vi "Check_Connectivity_111-11_with_101_Subtracks-1.vi"(4 "[IN] Index of connected tracks \nwith \"101\" problem dot":i32[](array[numeric]), 6 "[IN] Index of connected tracks \nwith \"111\" or \"11\" problem dot":i32[](array[numeric])) -> (1 "[OUT] Tracks aren't \nconnected after \"101\"":bool)   [LabVIEW 2013]
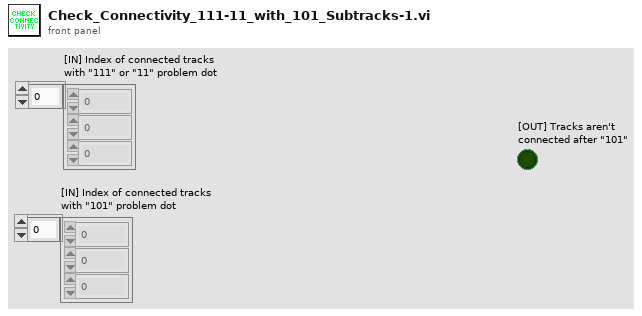
[diagram p1: front panel]
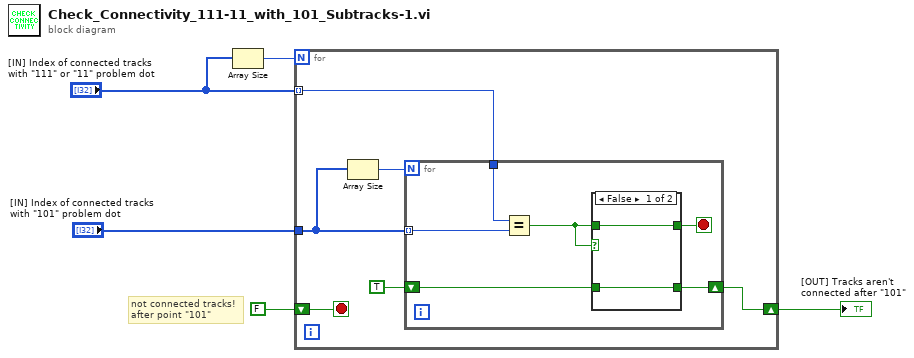
[diagram p0: block diagram]
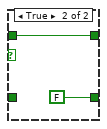
[diagram p2: hidden frame]
diagram:
  # "not connected tracks!\nafter point \"101\""
  n1 = Array Size(array="[IN] Index of connected tracks \nwith \"111\" or \"11\" problem dot") -> (size(s)=w5:i32)
  n2 = for {
    N: w5 -> [_]
    tunnel: "[IN] Index of connected tracks \nwith \"111\" or \"11\" problem dot" -> [w10] mode=indexing
    shift-right: [w6] -> w1
    shift-left: FALSE -> [w8]
    tunnel: "[IN] Index of connected tracks \nwith \"101\" problem dot" -> [w9]
    stop <- w8 stop-if-true
    n3 = Array Size(array=w9) -> (size(s)=w11:i32)
    n4 = for {
      N: w11 -> [_]
      tunnel: w9 -> [w17] mode=indexing
      tunnel: w10 -> [w16]
      shift-right: [w13] -> w6
      shift-left: TRUE -> [w14]
      stop <- w15 stop-if-true
      n5 = Equal?(x=w16, y=w17) -> (x = y?=w12:bool)
      n6 = case shown="False" w12 {
        tunnel: w12 -> [w19 w21]
        tunnel: [w19 w21] -> w15
        tunnel: w14 -> [w18 _]
        tunnel: [w18 FALSE] -> w13
        frame False {
        }
        frame True {
        }
      }
    }
  }
  "[OUT] Tracks aren't \nconnected after \"101\"" <- w1
